vi "Begin.vi"(8 "error in":errorcluster) -> (0 "error out":errorcluster)   [LabVIEW 2018]
doc: "Called before other user functions, this VI is expected to open initial I/O refnums, load in file data, and do all program initialization. Notice that the <B>error out</B> terminal is simply used for data flow. Wiring it to other structures or subVIs ensures that this VI runs first."
uses:
  <vilib>/Rock Robotics/WPI/DriverStation/WPI_DriverStationRobotMode2.ctl
  Global_Variables/Robot_Global_Data.vi
  <vilib>/Rock Robotics/Network Tables/NT Write String.vi
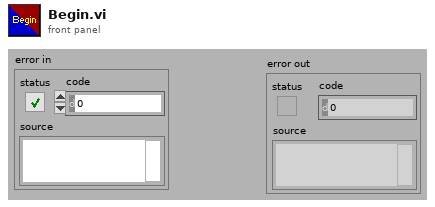
[diagram p1: front panel]
types:
  T1 = typedef "WPI_DriverStationRobotMode2.ctl" = enum16{"Autonomous Disabled", "Autonomous Enabled", "Teleop Disabled", "Teleop Enabled", "Disconnected", "Finish", "Test Disabled", "Test Enabled", "Emergency Stopped"}
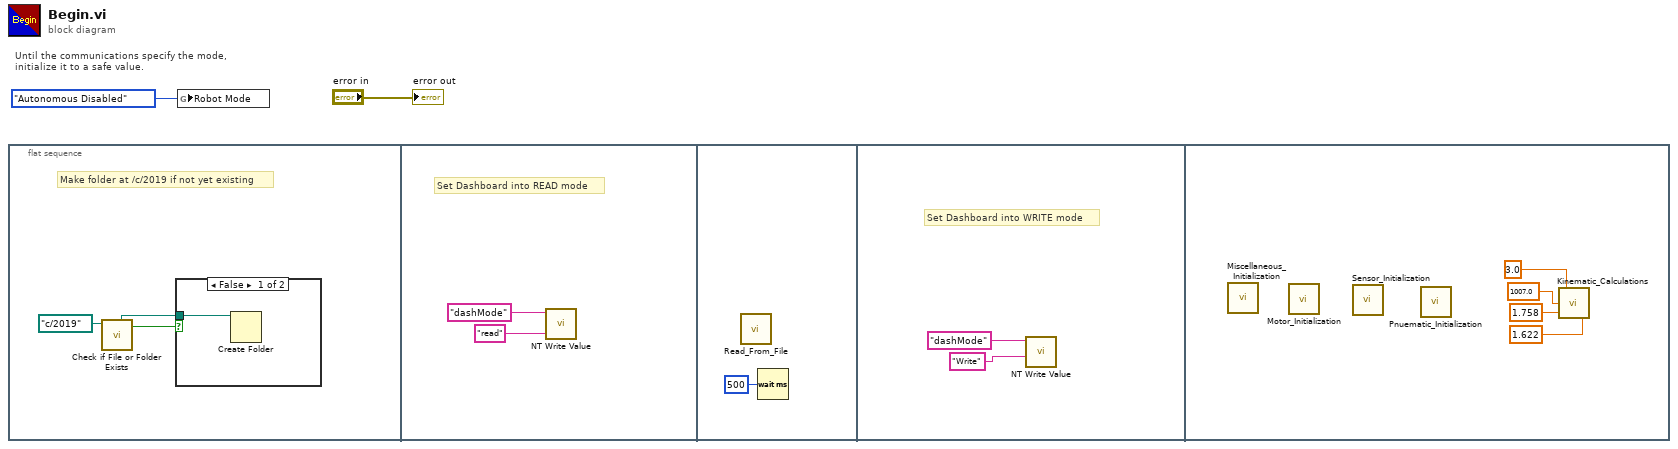
[diagram p0: block diagram]
diagram:
  # "Until the communications specify the mode,\ninitialize it to a safe value."
  n1 = flat-sequence {
    frame #0 {
      # "Make folder at /c/2019 if not yet existing"
      n2 = call <vilib>:"Check if File or Folder Exists.vi"("path"=path "c:/2019") -> ("file or folder exists?"=w5:bool, "dup path"=w3:path)  [unwired: 8 in, 1 out]
      n3 = case shown="False" w5 {
        tunnel: w3 -> [w6 _]
        frame False {
          n4 = Create Folder(path (use dialog)=w6) -> ()  [unwired: 2 in, 3 out]
        }
        frame True {
        }
      }
    }
    frame #1 {
      # "Set Dashboard into READ mode"
      n5 = call-poly <vilib>:"NT Write Value.vi"("String"="read", "Name"="dashMode") -> ()  [unwired: 9 in, 1 out]
    }
    frame #2 {
      n6 = call "Read_From_File.vi"() -> ()  [unwired: 12 in]
      n7 = Wait (ms)(milliseconds to wait=u32 500) -> ()  [unwired: 1 out]
    }
    frame #3 {
      # "Set Dashboard into WRITE mode"
      n8 = call-poly <vilib>:"NT Write Value.vi"("String"="Write", "Name"="dashMode") -> ()  [unwired: 9 in, 1 out]
    }
    frame #4 {
      n9 = call "Miscellaneous_Initialization.vi"() -> ()  [unwired: 12 in]
      n10 = call "Motor_Initialization.vi"() -> ()  [unwired: 12 in]
      n11 = call "Sensor_Initialization.vi"() -> ()  [unwired: 12 in]
      n12 = call "Pnuematic_Initialization.vi"() -> ()  [unwired: 12 in]
      n13 = call "Kinematic_Calculations.vi"("Width (ft)"=1.622, "Length (ft)"=1.758 ("Side_Length (ft)"), "Max_Wheel_Speed (rpm)"=1007.0, "Wheel_Diamater (in)"=3.0) -> ()  [unwired: 1 in]
    }
  }
  n14 = global write "Robot_Global_Data.vi" "Robot Mode"(WPI_DriverStationRobotMode2."Autonomous Disabled" ("Robot Mode")) -> ()
  "error out" <- "error in"
